vi "MAVLink CRC v2 Check.vi"(11 "Message":u8[](array[numeric]) format="%x") -> (3 "CRC good":bool)   [LabVIEW 2014]
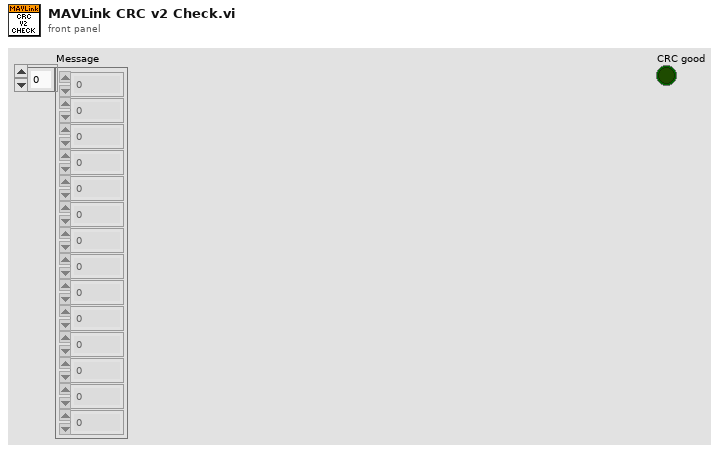
[diagram p1: front panel]
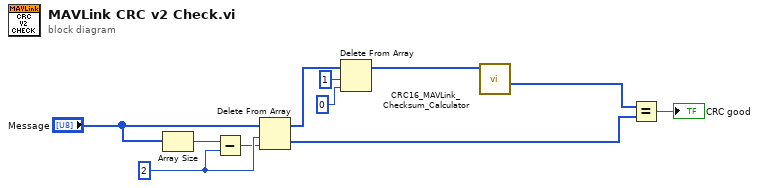
[diagram p0: block diagram]
diagram:
  w9 = 2 ("y")
  n1 = Array Size(array="Message") -> (size(s)=w10:i32)
  n2 = Subtract(x=w10, y=w9) -> (x-y=w8:i32)
  n3 = Delete From Array(array="Message", length=w9, index=w8) -> (deleted portion=w2:u8[], array with subset deleted=w7:u8[])
  n4 = Delete From Array(array=w7, length=1, index=0) -> (array with subset deleted=w4:u8[])  [unwired: 1 out]
  n5 = call "CRC16_MAVLink_Checksum_Calculator.vi"("Message"=w4) -> ("Bytes"=w3:u8[])  [unwired: 9 in, 1 out]
  n6 = Equal?(x=w3, y=w2) -> (x = y?=→"CRC good":bool)
